vi "SerialPortInit.vi"(8 "错误输入":errorcluster caption="错误输入（无错误）", 10 "海马":bool, 11 "COMIn":refnum<visa-resource-name>="COM1") -> (0 "错误输出":errorcluster, 3 "COMOut":refnum<visa-resource-name>)   [LabVIEW 2013]
uses:
  C:/Program Files/National Instruments/LabVIEW 2013/examples/Instrument IO/Serial/support/Serial - Settings.ctl
  <vilib>/Instr/_visa.llb/VISA Flush IO Buffer Mask.ctl
  <vilib>/Instr/_visa.llb/VISA Configure Serial Port (Instr).vi
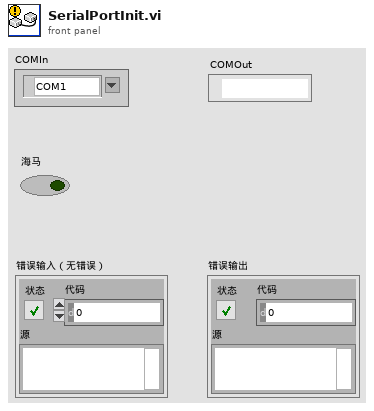
[diagram p1: front panel]
types:
  T1 = typedef "Serial - Settings.ctl" = cluster{"波特率":u32, "数据比特":u16, "奇偶":enum16{"None", "Odd", "Even", "Mark", "Space"}, "停止位":u16, "流控制":u16}
  T2 = typedef "VISA Flush IO Buffer Mask.ctl" = u16
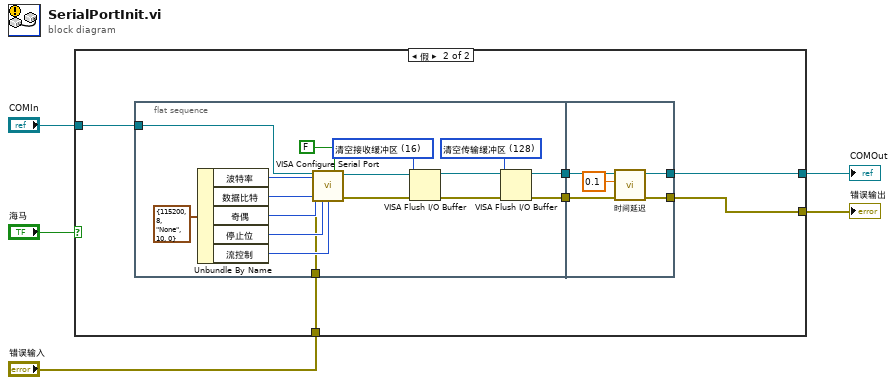
[diagram p0: block diagram]
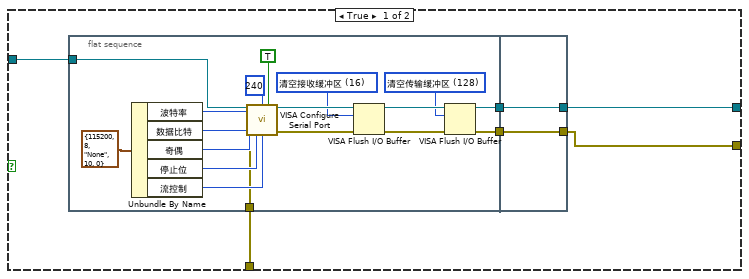
[diagram p2: hidden frame]
diagram:
  n1 = case shown="假" "海马" {
    tunnel: [w9 w36] -> w5
    tunnel: [w8 w35] -> w4
    tunnel: "错误输入" -> [w7 w34]
    tunnel: "COMIn" -> [w6 w33]
    frame True {
      n2 = flat-sequence {
        tunnel: w7 -> [w23]
        tunnel: [w17] -> w11
        tunnel: [w16] -> w10
        tunnel: w6 -> [w20]
        tunnel: [w30] -> w9
        tunnel: [w31] -> w8
        tunnel: w11 -> [w31]
        tunnel: w10 -> [w30]
        frame #0 {
          w12 = T2 128 items=["清空接收缓冲区"=16, "向设备写入传输缓冲区"=32, "清空接收缓冲区（无I/O）"=64, "清空传输缓冲区"=128] ("Mask")
          w13 = T2 16 items=["清空接收缓冲区"=16, "向设备写入传输缓冲区"=32, "清空接收缓冲区（无I/O）"=64, "清空传输缓冲区"=128] ("Mask")
          n3 = Unbundle By Name(T1 {"波特率"=115200, "数据比特"=8, "奇偶"=enum."None", "停止位"=10, "流控制"=0} ("串口设置")) -> ("波特率"=w26:u32, "数据比特"=w27:u16, "奇偶"=w28:enum16{"None", "Odd", "Even", "Mark", "Space"}, "停止位"=w29:u16, "流控制"=w24:u16)
          n4 = call-poly "VISA Configure Serial Port"("VISA resource name"=w20, "termination char\n(0xA = '\\n' = LF)"=u8 240 ("termination char\n(0xA = '\\n' = LF)"), "Enable Termination\nChar (T)"=TRUE ("Enable Termination\nChar (T)"), "baud rate (9600)"=w26, "data bits (8)"=w27, "parity (0:none)"=w28, "error in (no error)"=w23, "stop bits (10: 1 bit)"=w29, "flow control (0:none)"=w24) -> ("VISA resource name out"=w14:refnum<visa-resource-name>, "error out"=w15:errorcluster)  [unwired: 1 in, 4 out]
          n5 = VISA Flush I/O Buffer(VISA resource name=w14, mask (16)=w13, error in (no error)=w15) -> (VISA resource name out=w18:refnum<visa-resource-name>, error out=w19:errorcluster)
          n6 = VISA Flush I/O Buffer(VISA resource name=w18, mask (16)=w12, error in (no error)=w19) -> (VISA resource name out=w17:refnum<visa-resource-name>, error out=w16:errorcluster)
        }
        frame #1 {
        }
      }
    }
    frame False {
      n7 = flat-sequence {
        tunnel: w34 -> [w48]
        tunnel: [w41] -> w37
        tunnel: w33 -> [w45]
        tunnel: [w40] -> w32
        tunnel: [w55] -> w36
        tunnel: [w56] -> w35
        tunnel: w37 -> [w56]
        tunnel: w32 -> [w57]
        frame #0 {
          w39 = T2 128 items=["清空接收缓冲区"=16, "向设备写入传输缓冲区"=32, "清空接收缓冲区（无I/O）"=64, "清空传输缓冲区"=128] ("Mask")
          w44 = T2 16 items=["清空接收缓冲区"=16, "向设备写入传输缓冲区"=32, "清空接收缓冲区（无I/O）"=64, "清空传输缓冲区"=128] ("Mask")
          n8 = Unbundle By Name(T1 {"波特率"=115200, "数据比特"=8, "奇偶"=enum."None", "停止位"=10, "流控制"=0} ("串口设置")) -> ("波特率"=w51:u32, "数据比特"=w52:u16, "奇偶"=w53:enum16{"None", "Odd", "Even", "Mark", "Space"}, "停止位"=w54:u16, "流控制"=w49:u16)
          n9 = call-poly "VISA Configure Serial Port"("VISA resource name"=w45, "Enable Termination\nChar (T)"=FALSE ("Enable Termination\nChar (T)"), "baud rate (9600)"=w51, "data bits (8)"=w52, "parity (0:none)"=w53, "error in (no error)"=w48, "stop bits (10: 1 bit)"=w54, "flow control (0:none)"=w49) -> ("VISA resource name out"=w46:refnum<visa-resource-name>, "error out"=w47:errorcluster)  [unwired: 2 in, 4 out]
          n10 = VISA Flush I/O Buffer(VISA resource name=w46, mask (16)=w44, error in (no error)=w47) -> (VISA resource name out=w42:refnum<visa-resource-name>, error out=w43:errorcluster)
          n11 = VISA Flush I/O Buffer(VISA resource name=w42, mask (16)=w39, error in (no error)=w43) -> (VISA resource name out=w41:refnum<visa-resource-name>, error out=w40:errorcluster)
        }
        frame #1 {
          n12 = call "时间延迟"("error in (no error)"=w57, "Delay Time (s)"=0.1) -> ("error out"=w55:errorcluster)  [unwired: 9 in]
        }
      }
    }
  }
  "错误输出" <- w5
  "COMOut" <- w4
